vi "SetMotors_with_PID(SUBVI(subvi)).vi"(10 "steering frame velocity":dbl[](array[numeric])=[0.0, 0.0, 0.0], 11 "Reset Encoders":bool) -> (1 "Taka":cluster{"initial PV":dbl, "SP:":dbl}(graph)={"initial PV"=0.0, "SP:"=-0.0}, 2 "Etu":cluster{"initial PV":dbl, "SP:":dbl}(graph)={"initial PV"=0.0, "SP:"=-0.0}, 3 "Radians/s":dbl[](array[numeric]), 4 "Vasen":cluster{"initial PV":dbl, "SP:":dbl}(graph)={"initial PV"=0.0, "SP:"=-0.0}, 5 "ccw motor velocity setpoints":dbl[](array[numeric])=[-0.0, -0.0, -0.0, -0.0], 6 "Oikea":cluster{"initial PV":dbl, "SP:":dbl}(graph)={"initial PV"=0.0, "SP:"=-0.0})   [LabVIEW 2018]
uses:
  <vilib>/robotics/Steering/Wheel/Wheel Parameters.ctl
  <vilib>/robotics/Steering/Wheel/Rotation Direction.ctl
  <vilib>/robotics/Steering/Omnidirectional Wheel/NI_Robotics_Omnidirectional Wheel.lvclass
  C:/Program Files (x86)/National Instruments/LabVIEW 2018/vi.lib/robotics/Steering/Wheel/NI_Robotics_Wheel.lvclass
  <vilib>/robotics/Steering/Omnidirectional Wheel/Create Omnidirectional Wheel.vi
  <vilib>/robotics/Steering/Steering Frame/Create User Defined Steering Frame.vi
  <vilib>/robotics/Steering/Steering Frame/Apply Steering Frame Velocity to Motors.vi
  <vilib>/addons/control/pid/pid.llb/PID (DBL Array).vi
  <vilib>/robotics/Steering/Create Steering Frame/NI_Robotics_Create Steering Frame.xnode
  <vilib>/robotics/Steering/Class Type Definitions/Steering Frame.ctl
  <vilib>/robotics/Steering/Steering Frame/NI_Robotics_Steering Frame.lvclass
  <vilib>/robotics/Steering/Class Type Definitions/NI_Robotics_Steering Class Types.lvlib
  <vilib>/robotics/Steering/Wheel/NI_Robotics_Wheel.lvclass
  <vilib>/addons/control/pid/NI_PID_pid.lvlib
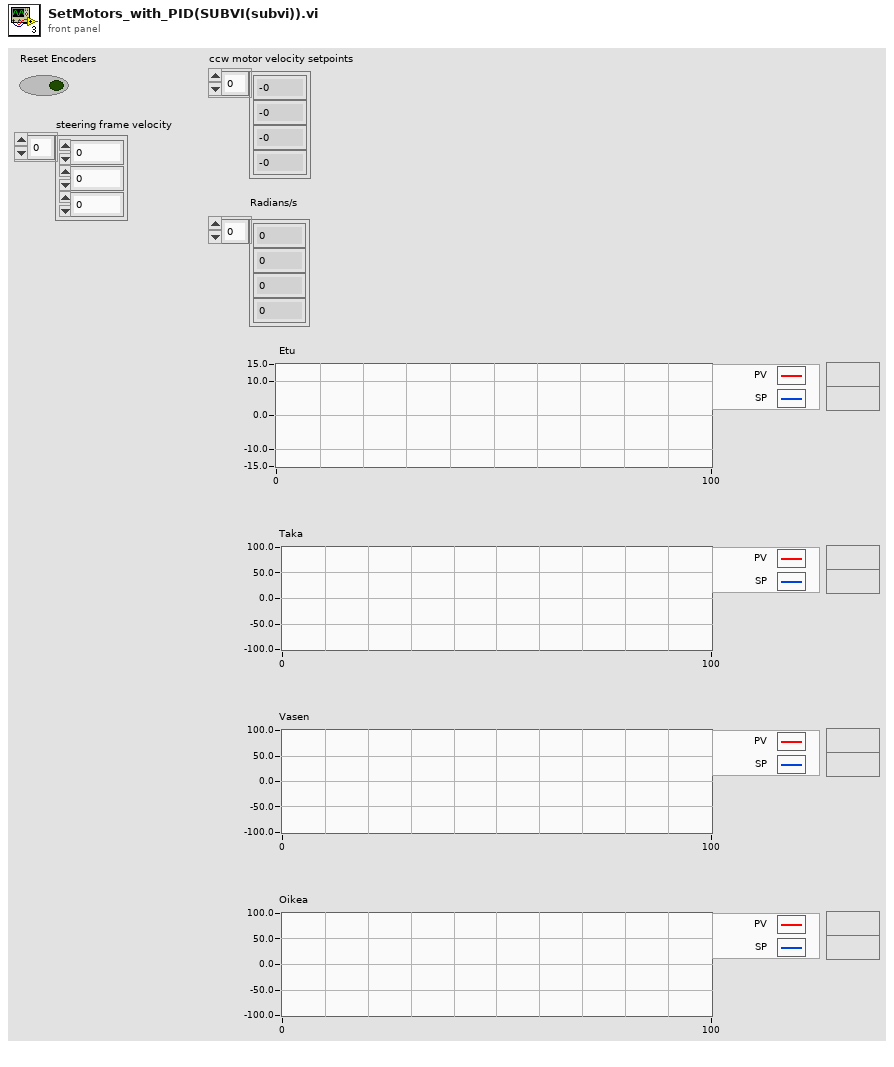
[diagram p1: front panel]
types:
  T1 = cluster{bool, "Tick Count(uSec)":u32, "Counter Value":i32[], "x-y":i32[]}
  T2 = typedef "NI_Robotics_Steering Class Types.lvlib/Steering Frame.ctl" = refnum<class "NI_Robotics_Steering Frame.lvclass">
  T3 = cluster{"Position":i32[], "Velocity RPM":dbl[], "Velocity RPS":dbl[], "Radians/s":dbl[]}
  T4 = cluster{"proportional gain (Kc)":dbl, "integral time (Ti, min)":dbl, "derivative time (Td, min)":dbl}[]
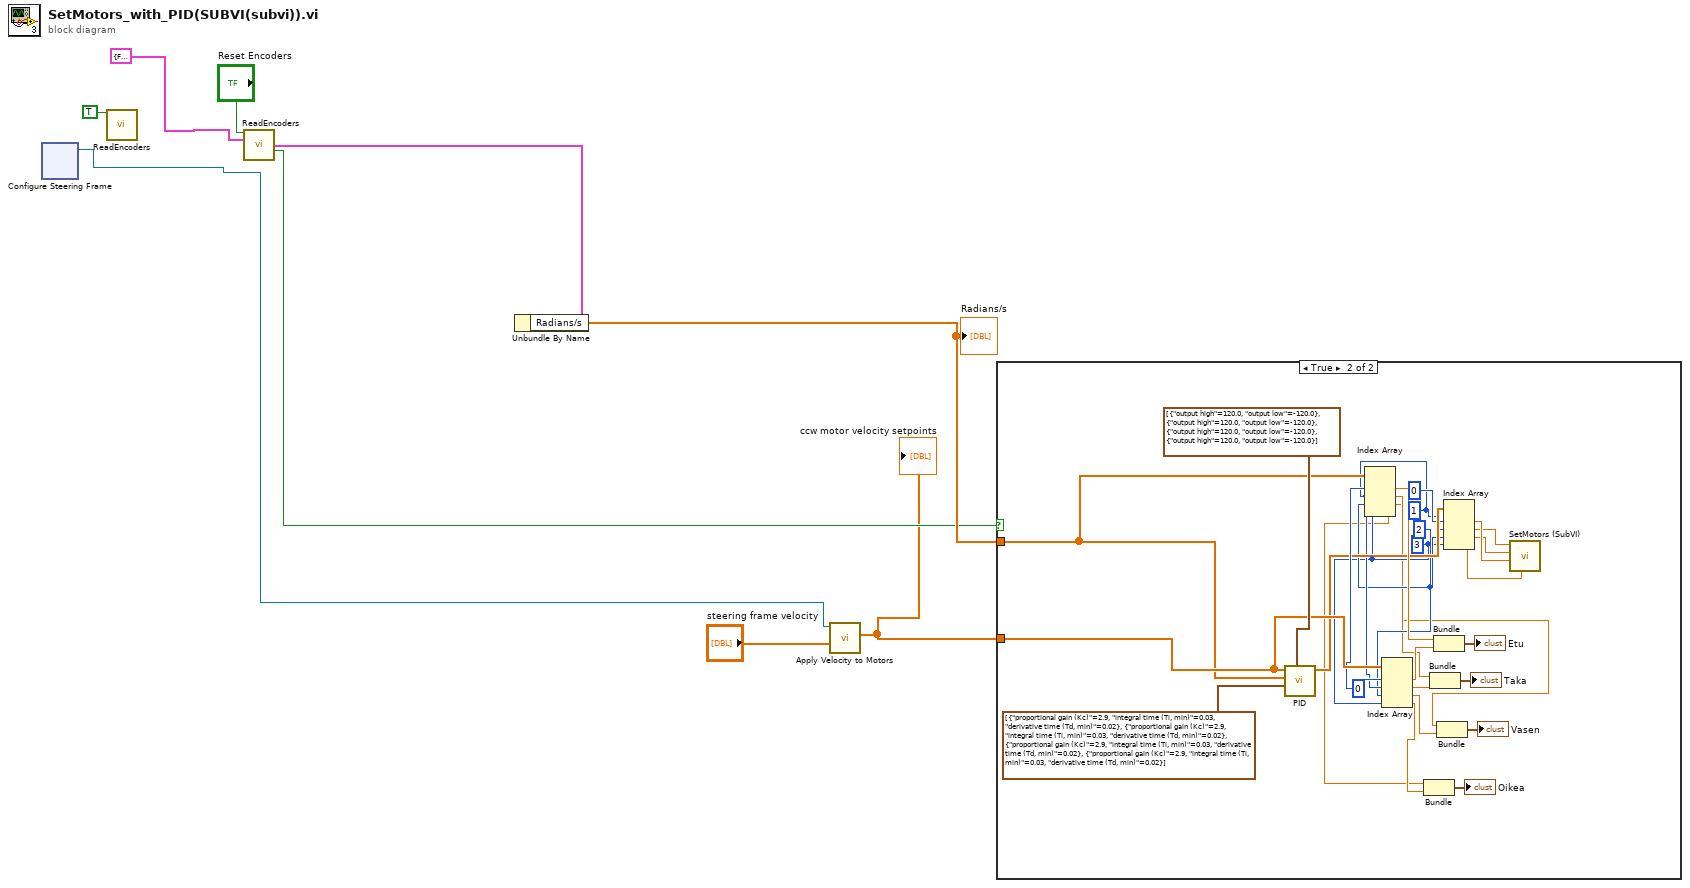
[diagram p0: block diagram]
diagram:
  n1 = xnode ("Configure Steering Frame")() -> ("steering frame out"=w2:T2)  [unwired: 1 in, 1 out]
  n2 = call "ReadEncoders.vi"("Reset Encoders"=TRUE) -> ()  [unwired: 10 in, 5 out]
  n3 = call "ReadEncoders.vi"("Reset Encoders"="Reset Encoders", "Cluster in"=T1 {FALSE, "Tick Count(uSec)"=0, "Counter Value"=[0, 0, 0, 0], "x-y"=[0, 0, 0, 0]}) -> ("output cluster"=w6:T3, "Updated"=w7:bool)  [unwired: 9 in, 3 out]
  n4 = Unbundle By Name(w6) -> ("Radians/s"=w8:dbl[])
  "Radians/s" <- w8
  n5 = call-poly <vilib>:"Apply Velocity to Motors.vi"("steering frame velocity"="steering frame velocity", "steering frame in"=w2) -> ("ccw motor velocity setpoints"=w5:dbl[])  [unwired: 5 in, 4 out]
  "ccw motor velocity setpoints" <- w5
  n6 = case shown="True" w7 {
    tunnel: w5 -> [_ w34]
    tunnel: w8 -> [_ w29]
    frame False {
    }
    frame True {
      w14 = 3 ("index")
      w15 = 2 ("index")
      w16 = 1 ("index")
      w33 = 0 ("index")
      n7 = call-poly <vilib>:"PID.vi"("output range"=cluster{"output high":dbl, "output low":dbl}[] [{"output high"=120.0, "output low"=-120.0}, {"output high"=120.0, "output low"=-120.0}, {"output high"=120.0, "output low"=-120.0}, {"output high"=120.0, "output low"=-120.0}], "PID gains"=T4 [{"proportional gain (Kc)"=2.9, "integral time (Ti, min)"=0.03, "derivative time (Td, min)"=0.02}, {"proportional gain (Kc)"=2.9, "integral time (Ti, min)"=0.03, "derivative time (Td, min)"=0.02}, {"proportional gain (Kc)"=2.9, "integral time (Ti, min)"=0.03, "derivative time (Td, min)"=0.02}, {"proportional gain (Kc)"=2.9, "integral time (Ti, min)"=0.03, "derivative time (Td, min)"=0.02}], "process variable"=w29, "setpoint"=w34) -> ("output"=w28:dbl[])  [unwired: 6 in, 1 out]
      n8 = Index Array(array=w29, index #1=w33, index #2=w16, index #3=w15, index #4=w14) -> (element #1=w31:dbl, element #2=w13:dbl, element #3=w12:dbl, element #4=w11:dbl)
      n9 = Index Array(array=w34, index #1=w33, index #2=w16, index #3=w15, index #4=w14) -> (element #1=w30:dbl, element #2=w17:dbl, element #3=w18:dbl, element #4=w19:dbl)
      n10 = Bundle(w11, "Numeric"=w19) -> (→"Oikea":cluster{dbl, "Numeric":dbl})  [unwired: 1 in]
      n11 = Bundle(w13, "Numeric"=w17) -> (→"Taka":cluster{dbl, "Numeric":dbl})  [unwired: 1 in]
      n12 = Bundle(w31, "Numeric"=w30) -> (→"Etu":cluster{dbl, "Numeric":dbl})  [unwired: 1 in]
      n13 = Bundle(w12, "Numeric"=w18) -> (→"Vasen":cluster{dbl, "Numeric":dbl})  [unwired: 1 in]
      n14 = Index Array(array=w28, index #1=0 ("index"), index #2=w16, index #3=w15, index #4=w14) -> (element #1=w26:dbl, element #2=w25:dbl, element #3=w24:dbl, element #4=w23:dbl)
      n15 = call "SetMotors (SubVI).vi"("Oikea"=w23, "Etu"=w26, "Vasen"=w24, "Taka"=w25) -> ()  [unwired: 8 in]
    }
  }
